vi "readmeterremotely_xw.vi"() -> ()   [LabVIEW 2015]
uses:
  Libraries/HeliumMonitor/Sensor configuration.ctl
  Libraries/HeliumMonitor/Channel type.ctl
  <vilib>/Platform/TimedLoop/XDataNode/timing_clust.ctl
  <vilib>/Platform/TimedLoop/XDataNode/nitl_modes.ctl
  <vilib>/Platform/TimedLoop/XDataNode/wakeup.ctl
  <vilib>/platform/TimedLoop/XDataNode/XDataNode.xnode
  <vilib>/Platform/TimedLoop/XDataNode/XDNodeRunTimeDep.lvlib
panel:
  out "Dewar level":i32(slide) scale=0.0..1000.0
  in  "Data Folder":path=path "\\\\eden\\NHMFLDATA/Data/nhmflmonitor/Helium/data"
  in  "Tab Control":T1(tab)
  out "History Graph":T2(graph)
  in  "Sensors":T3[](array[typedef])=[{"Name"="Ghz lab", "URL"="http:\\\\130.55.69.25", "Channels"=[{"type"=enum."Flow meter", "number"=6.0}]}, {"Name"="main bag", "URL"="http:\\\\130.55.69.22", "Channels"=[{"type"=enum."Flow meter", "number"=6.0}, {"type"=enum."Tank pressure", "number"=0.0}, {"type"=enum."Dewar level", "number"=1.0}]}, {"Name"="PPMS 20T", "URL"="http:\\\\130.55.69.42", "Channels"=[{"type"=enum."Flow meter", "number"=6.0}]}]
  out "Communication Status":string[](array[string])
  in  "Ignore errors":bool
  out "Helium tank pressure":dbl(knob) scale=0.0..2000.0
  in  "period (ms)":i32=5000
  in  "Display Graph":bool=TRUE
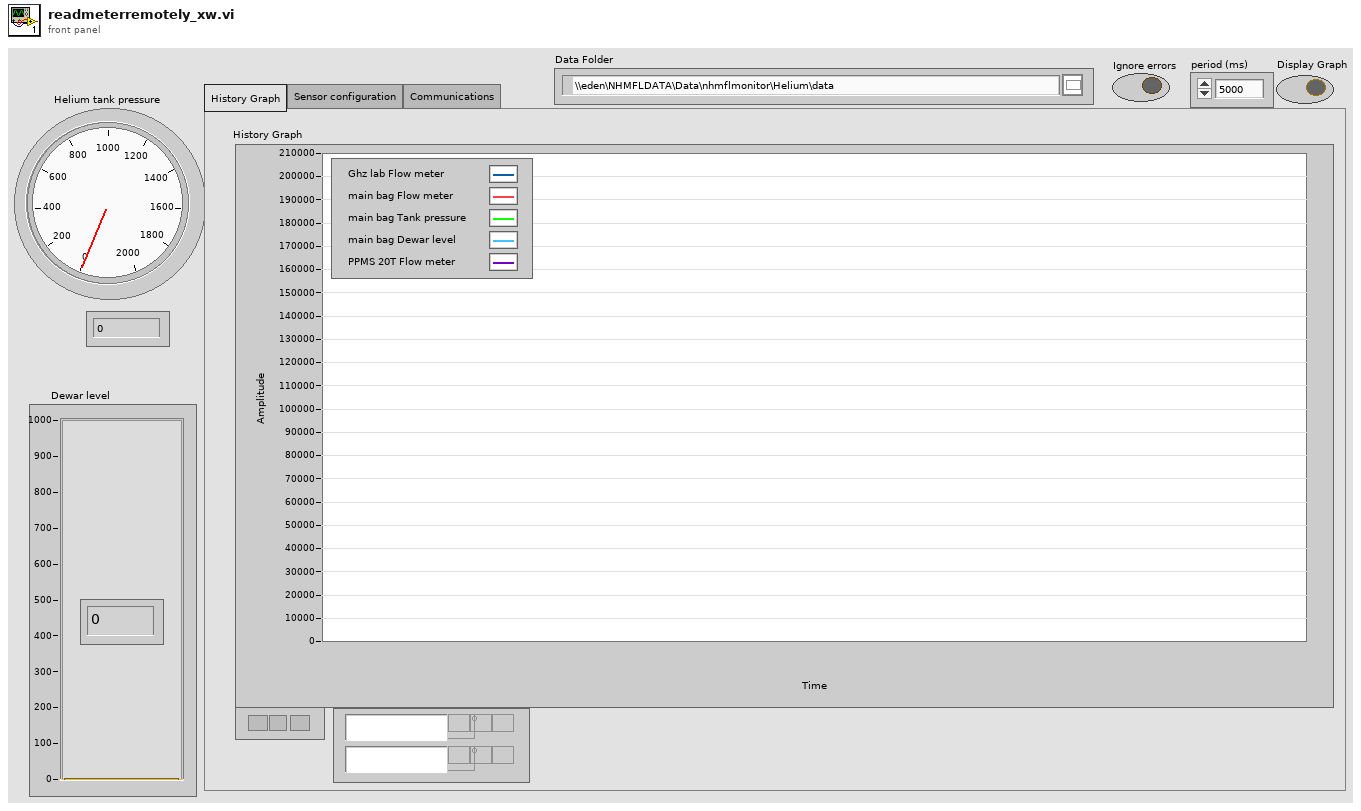
[diagram p1: front panel]
types:
  T1 = enum32{"History Graph", "Sensor configuration", "Communications"}
  T2 = cluster{"output array":dbl[], "output array":dbl[]}[]
  T3 = typedef "Sensor configuration.ctl" = cluster{"Name":string, "URL":string, "Channels":cluster{"type":T4, "number":dbl}[]}
  T4 = typedef "Channel type.ctl" = enum16{"Volts", "Flow meter", "Tank pressure", "Dewar level", "Raw ADC"}
  T5 = typedef "XDNodeRunTimeDep.lvlib/timing_clust.ctl" = cluster{"Expected End [f-1]":u64, "Actual End [f-1]":u64, "Finished Late? [f-1]":bool, "Expected End [i-1]":u64, "Actual End [i-1]":u64, "Finished Late? [i-1]":bool, "Expected Start [i]":u64, "Actual Start [i]":u64, "Expected Start [f]":u64, "Actual Start [f]":u64, "Source Name":string, "Structure Name":string, "Period":i64, "Deadline":i64, "Offset":i64, "Start":i64, "Priority":i32, "Timeout":i32, "Mode":T6, "Wakeup Reason":T7, "Error":errorcluster, "Source Type":string, "Secondary Source Type":string, "Global End Time":u64, "Global Start Time":u64, "Frame Duration":u64, "Iteration Duration":u64, "Assigned CPU":i32, "I/O Scan Engine Mode":u32}
  T6 = typedef "XDNodeRunTimeDep.lvlib/nitl_modes.ctl" = enum32{"No Change", "Process missed periods, maintain original phase", "Discard missed periods, maintain original phase", "Process missed periods, ignore original phase", "Discard missed periods, ignore original phase"}
  T7 = typedef "XDNodeRunTimeDep.lvlib/wakeup.ctl" = enum32{"Normal", "Aborted", "Asynchronous wakeup", "Timing source error", "Timed loop error", "Timeout"}
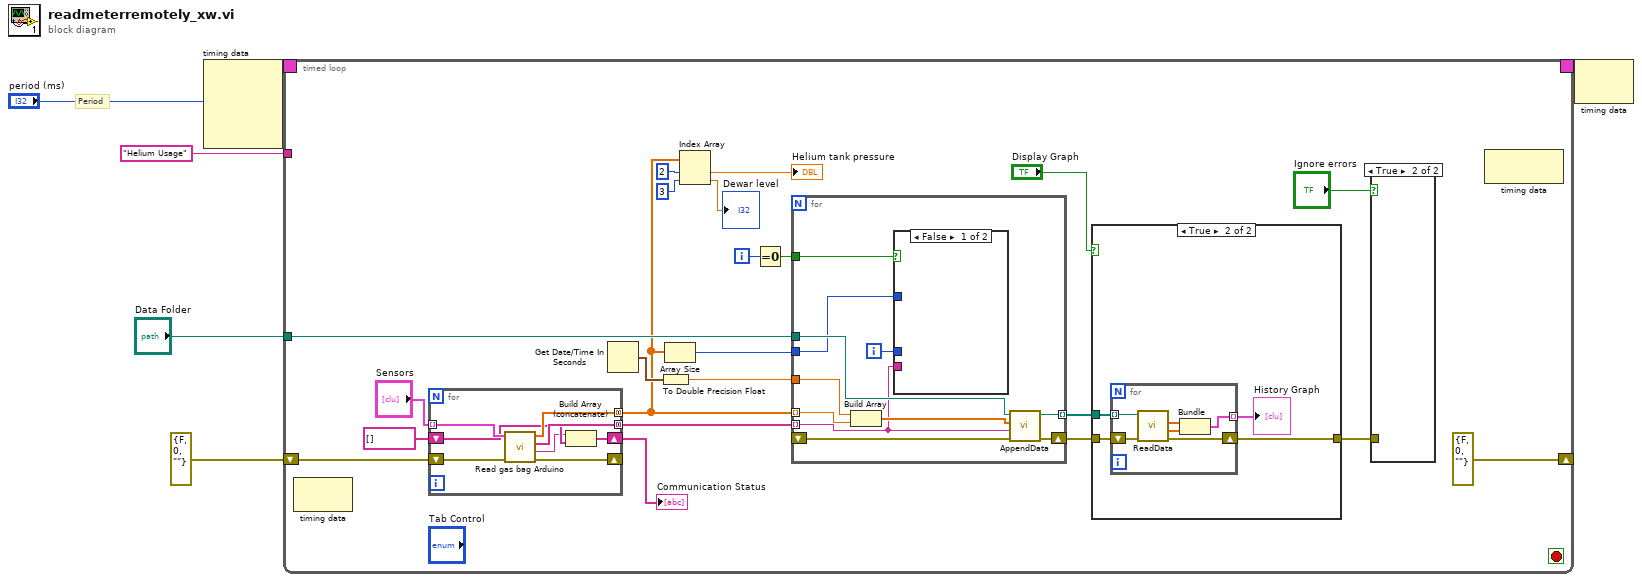
[diagram p0: block diagram]
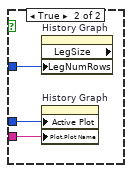
[diagram p2: hidden frame]
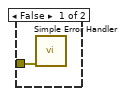
[diagram p3: hidden frame]
diagram:
  # "Period"
  n1 = node-c288("period (ms)") -> (w6:T5)  [unwired: 3 in]
  n2 = timed-loop {
    timing: w6 -> [_]
    timing-out: [_] -> w5
    tunnel: "Data Folder" -> [w15]
    tunnel: "Helium Usage" -> [_]
    shift-right: [errorcluster {"status"=FALSE, "code"=0, "source"=""} ("error out")] -> _
    shift-left: errorcluster {"status"=FALSE, "code"=0, "source"=""} ("error out") -> [w25]
    i -> [w13]
    stop <- _ stop-if-true
    n3 = node-c288() -> ()  [unwired: 1 in, 1 out]
    n4 = for {
      tunnel: "Sensors" -> [w50] mode=indexing
      shift-right: [w47] -> _
      shift-left: w25 -> [w51]
      tunnel: [w49] -> w10 mode=concatenating
      tunnel: [w48] -> w19 mode=concatenating
      shift-right: [w46] -> w7
      shift-left: string[] [] -> [w45]
      n5 = call "Read gas bag Arduino.vi"("Sensor configuration"=w50, "Error In"=w51) -> ("Data"=w49:dbl[], "Names"=w48:string[], "Communication error"=w44:string, "Error Out"=w47:errorcluster)  [unwired: 5 in]
      n6 = Build Array (concatenate)(w44, w45) -> (w46:string[])
    }
    "Communication Status" <- w7
    n7 = Get Date/Time In Seconds() -> (seconds since 1Jan1904=w27:timestamp)
    n8 = To Double Precision Float(number=w27) -> (double precision float=w20:dbl)
    n9 = Array Size(array=w10) -> (size(s)=w9:i32)
    n10 = Index Array(array=w10, index #1=2 ("index"), index #2=3 ("index")) -> (element #1=→"Helium tank pressure":dbl, element #2=→"Dewar level":dbl)
    n11 = Equal To 0?(x=w13) -> (x = 0?=w12:bool)
    n12 = for {
      tunnel: w10 -> [w35] mode=indexing
      shift-right: [w38] -> w26
      shift-left: _ -> [w37]
      tunnel: w20 -> [w36]
      tunnel: w19 -> [w31] mode=indexing
      tunnel: w15 -> [w39]
      tunnel: [w33] -> w14 mode=indexing
      tunnel: w12 -> [w30]
      tunnel: w9 -> [w29]
      i -> [w32]
      n13 = Build Array(w36, w35) -> (w34:dbl[])
      n14 = case shown="False" w30 {
        tunnel: w32 -> [_ w42]
        tunnel: w31 -> [_ w41]
        tunnel: w29 -> [_ w40]
        frame False {
        }
        frame True {
          n15 = property on="History Graph" class="XYGraph (strict)" props=["LegSize", "LegNumRows"]("LegNumRows"=w40) -> ()  [unwired: 2 in, 3 out]
          n16 = property on="History Graph" class="XYGraph (strict)"("Active Plot"=w42, "Plot.Plot Name"=w41) -> ()  [unwired: 2 in, 2 out]
        }
      }
      n17 = call "AppendData.vi"("Error In"=w37, "Name"=w31, "Data"=w34, "Folder"=w39) -> ("Error Out"=w38:errorcluster, "File Path Control out"=w33:path)  [unwired: 6 in]
    }
    n18 = case shown="True" "Display Graph" {
      tunnel: w14 -> [_ w53]
      tunnel: w26 -> [w52 w56]
      tunnel: [w52 w55] -> w23
      frame False {
      }
      frame True {
        n19 = for {
          shift-right: [w61] -> w55
          shift-left: w56 -> [w62]
          tunnel: [w60] -> w54 mode=indexing
          tunnel: w53 -> [w57] mode=indexing
          n20 = call "ReadData.vi"("Error In"=w62, "File Path Control"=w57) -> ("Error Out"=w61:errorcluster, "Y"=w58:dbl[], "X"=w59:dbl[])  [unwired: 6 in, 1 out]
          n21 = Bundle("X"=w59, "Y"=w58) -> (w60:cluster{"X":dbl[], "Y":dbl[]})  [unwired: 1 in]
        }
        "History Graph" <- w54
      }
    }
    n22 = case shown="True" "Ignore errors" {
      tunnel: w23 -> [w43 _]
      frame False {
        n23 = call <vilib>:"Simple Error Handler.vi"("error in (no error)"=w43) -> ()  [unwired: 4 in, 5 out]
      }
      frame True {
      }
    }
    n24 = node-c288() -> ()  [unwired: 1 in, 1 out]
  }
  n25 = node-c288(w5) -> ()  [unwired: 1 out]
